vi "dialog box.vi"(1 "Status":string="Warning:\nTrained and authorized users only! \nEnsure all positioners are tightened and specimens are mounted securely.\nMoving machinery can cause serious injuries - keep away when equipment is in operation. \n", 3 "error in":errorcluster) -> (10 "error out":errorcluster)   [LabVIEW 2025]
panel:
  in  "Boolean":bool
  in  "OK":bool
  # "Warning:\nTrained and authorized users only! Ensure all positioners are tightened and specimens are mounted securely.\nMoving machinery can cause serious injuries - keep away when equipment is in operation."
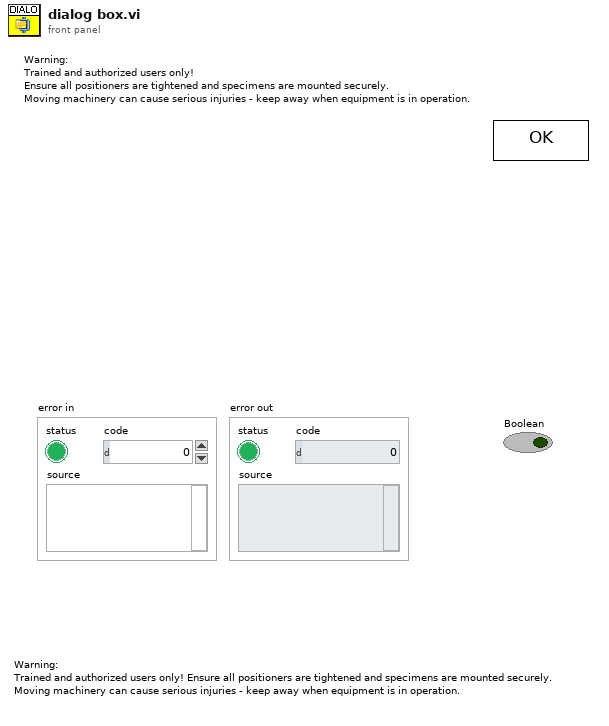
[diagram p1: front panel]
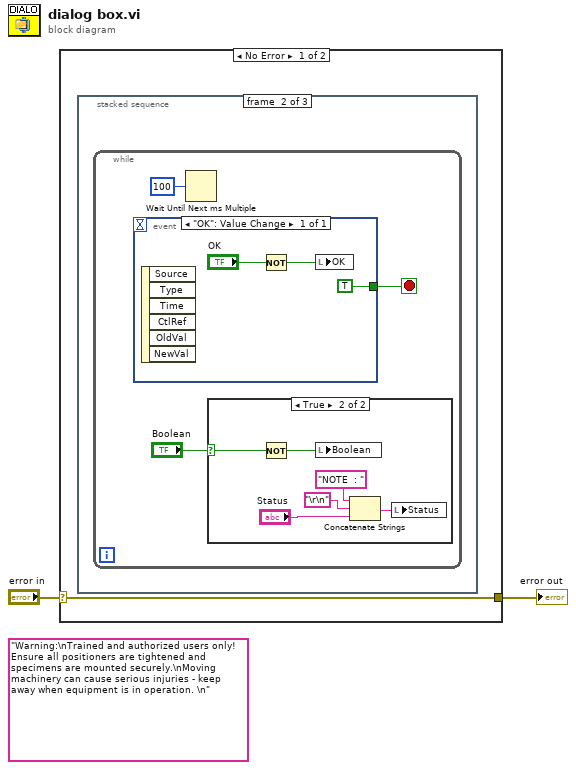
[diagram p0: block diagram]
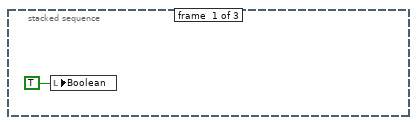
[diagram p2: hidden frame]
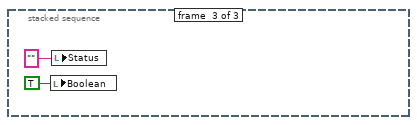
[diagram p4: hidden frame]
diagram:
  (unwired) "Warning:\nTrained and authorized users only! Ensure all positioners are tightened and specimens are mounted securely.\nMoving machinery can cause serious injuries - keep away when equipment is in operation. \n" ("message")
  n1 = case shown="No Error" "error in" {
    selector: "error in" -> [w3 _]
    tunnel: [w3 _] -> w1
    frame No Error {
      n2 = stacked-sequence {
        frame #0 {
          n3 = local write "Boolean"(TRUE ("Boolean")) -> ()
        }
        frame #1 {
          n4 = while {
            stop <- w6 stop-if-true
            n5 = event shown="[0] \"OK\": Value Change" {
              selector: _ -> [_]
              dyn-events: _ -> [_]
              timeout: _ -> [_]
              tunnel: [TRUE] -> w6
              event "OK": Value Change {
                n6 = event-data() -> ()  [unwired: 1 in, 6 out]
                n7 = Not(x="OK") -> (.not. x?=w14:bool)
                n8 = local write "OK"(w14) -> ()
              }
            }
            n9 = Wait Until Next ms Multiple(millisecond multiple=100) -> ()  [unwired: 1 out]
            n10 = case shown="True" "Boolean" {
              selector: "Boolean" -> [_ w12]
              frame False {
              }
              frame True {
                n11 = Not(x=w12) -> (.not. x?=w11:bool)
                n12 = local write "Boolean"(w11) -> ()
                n13 = Concatenate Strings("NOTE  : ", "\r\n", "Status") -> (w10:string)
                n14 = local write "Status"(w10) -> ()
              }
            }
          }
        }
        frame #2 {
          n15 = local write "Boolean"(TRUE ("Boolean")) -> ()
          n16 = local write "Status"("") -> ()
        }
      }
    }
    frame Error {
    }
  }
  "error out" <- w1
